vi "Ex1_Add_COM_Array.vi"() -> ()   [LabVIEW 2013]
panel:
  out "Array Sum":dbl[](array[numeric])
  in  "Array b":dbl[](array[numeric])
  in  "Array a":dbl[](array[numeric])
  in  "Ex1_add.IClass1":refnum<k7>
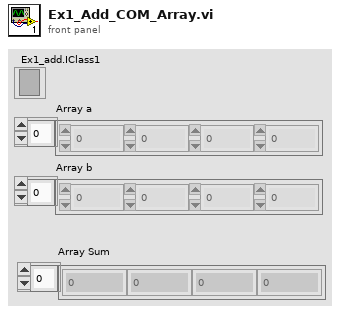
[diagram p1: front panel]
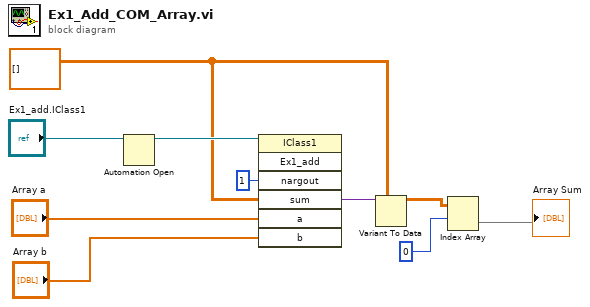
[diagram p0: block diagram]
diagram:
  w4 = dbl[][] []
  n1 = Automation Open(Automation Refnum="Ex1_add.IClass1") -> (Automation Refnum=w9:refnum<k7>)  [unwired: 3 in, 1 out]
  n2 = invoke class="IClass1" method="Ex1_add"(reference=w9, "nargout"=1, "sum"=w4, "a"="Array a", "b"="Array b") -> ("sum"=w8:variant)  [unwired: 2 in, 6 out]
  n3 = Variant To Data(type=w4, Variant=w8) -> (data=w3:dbl[][])  [unwired: 1 in, 1 out]
  n4 = Index Array(array=w3, index (row)=0) -> (element=→"Array Sum":dbl[])  [unwired: 1 in]
